vi "Configure Input Impedance.vi"(8 "error in (no error)":errorcluster, 10 "Input Impedance Mode (0: Fixed)":u16(ring) items=["Fixed", "Auto"], 11 "VISA resource name":refnum<visa-resource-name>) -> (0 "error out":errorcluster, 3 "VISA resource name out":refnum<visa-resource-name>)   [LabVIEW 2010, in "Fluke 884X Series.lvlib"]
doc: "Sets the input impedance for voltage readings."
uses:
  <instrlib>/Fluke 884X Series/Fluke 884X Series.lvlib
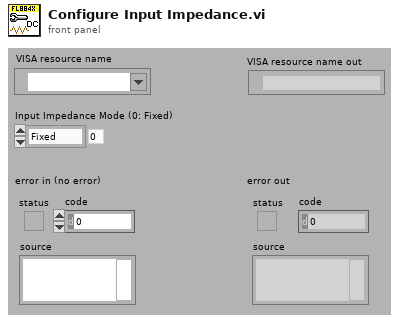
[diagram p1: front panel]
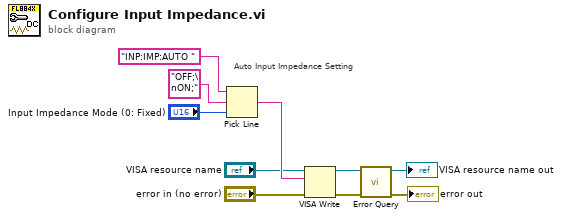
[diagram p0: block diagram]
diagram:
  # "Auto Input Impedance Setting"
  n1 = Pick Line(string ("")="INP:IMP:AUTO ", multi-line string="OFF;\nON;", line index="Input Impedance Mode (0: Fixed)") -> (output string=w10:string)
  n2 = VISA Write(VISA resource name="VISA resource name", write buffer=w10, error in (no error)="error in (no error)") -> (VISA resource name out=w8:refnum<visa-resource-name>, error out=w9:errorcluster)  [unwired: 1 out]
  n3 = call <instrlib>:"Error Query.vi"("error in (no error)"=w9, "VISA resource name"=w8) -> ("error out"=→"error out":errorcluster, "VISA resource name out"=→"VISA resource name out":refnum<visa-resource-name>)  [unwired: 6 in, 2 out]
